vi "Acquiring a Signal.vi"() -> ()   [LabVIEW 2016]
doc: "Use this template to simulate the generation and display of data.\nNote: LabVIEW enables automatic error handling by default for VIs you create from this template."
uses:
  Instance           1 27Saved   GenerateDisplay.vit .vi
  <vilib>/express/express shared/transition.llb/Dynamic To Waveform Array.vi
  <vilib>/express/express arith-compare/Formula/Block/exnFormulaBlock how many pts in the wave.vi
  <vilib>/express/express shared/ex_Modify Signal Name.vi
  <vilib>/express/express shared/transition.llb/Waveform Array To Dynamic.vi
  <vilib>/express/express arith-compare/Formula/XNode/ExpressFormulaBlockNode.xnode
panel:
  in  "Amplitude":dbl(knob) scale=0.0..10.0
  out "Waveform Graph":dynamicdata(graph)
  in  "stop":bool
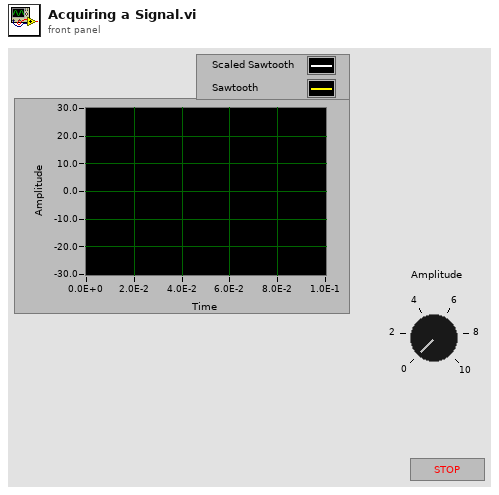
[diagram p1: front panel]
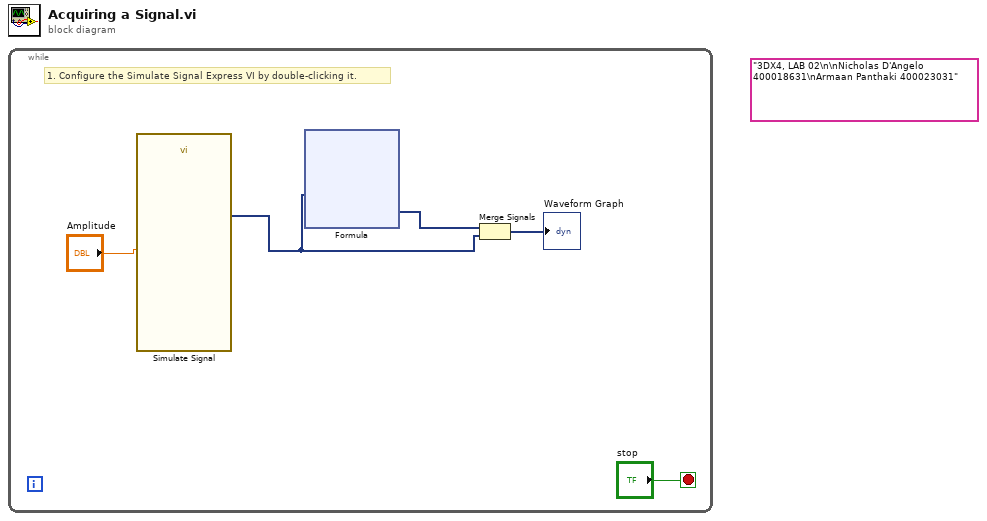
[diagram p0: block diagram]
diagram:
  (unwired) "3DX4, LAB 02\n\nNicholas D'Angelo 400018631\nArmaan Panthaki 400023031"
  n1 = while {
    stop <- "stop" stop-if-true
    # "1. Configure the Simulate Signal Express VI by double-clicking it."
    n2 = call "Simulate Signal"("Amplitude"="Amplitude") -> ("Sawtooth"=w1:dynamicdata)  [unwired: 13 in, 1 out]
    n3 = xnode "Formula"("Sawtooth"=w1) -> ("Result"=w3:dynamicdata)  [unwired: 1 in, 1 out]
    n4 = Merge Signals(w3, w1) -> (→"Waveform Graph":dynamicdata)
  }
